vi "Open Adu Stream.vi"(7 "Timeout":u32, 8 "error in (no error)":errorcluster) -> (0 "error out":errorcluster, 3 "function return":u32)   [LabVIEW 2015, in "AduHid.lvlib"]
doc: "void * __stdcall OpenAduStream(unsigned long iTimeout);"
uses:
  AduHid.lvlib
  AduHid.dll
  Windows/SysWOW64/kernel32.dll
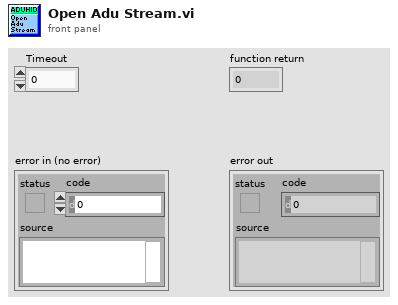
[diagram p1: front panel]
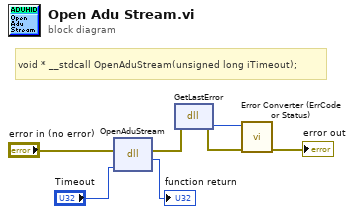
[diagram p0: block diagram]
diagram:
  # "void * __stdcall OpenAduStream(unsigned long iTimeout);"
  n1 = dll-call lib="C:/Projects/CBTF Modules/Libraries/Ontrak ADU/API/AduHid.*" fn="OpenAduStream"(error in="error in (no error)", "Timeout"="Timeout") -> (error out=w2:errorcluster, "return type"=→"function return":u32)  [unwired: 3 in, 1 out]
  n2 = dll-call lib="C:/Windows/SysWOW64/kernel32.dll" fn="GetLastError"(error in=w2) -> (error out=w4:errorcluster, "return type"=w3:u32)  [unwired: 2 in, 1 out]
  n3 = call "Error Converter (ErrCode or Status).vi"("error in (no error)"=w4, "last error"=w3) -> ("error out"=→"error out":errorcluster)  [unwired: 9 in]
